vi "plot_normal.vi"(0 "mean":dbl, 1 "standard deviation":dbl, 2 "variance":dbl, 5 "error in (no error)":errorcluster, 6 "xsup":dbl, 8 "xinf":dbl, 10 "N":u16) -> (14 "Normal_xy":cluster{dbl[], dbl[]}, 15 "x":dbl[](array[numeric]), 16 "Normal curve":dbl[](array[numeric]), 19 "error out":errorcluster)   [LabVIEW 2019]
panel:
  in  "Tab Control":enum32{"Page 1", "Page 2"}(tab)
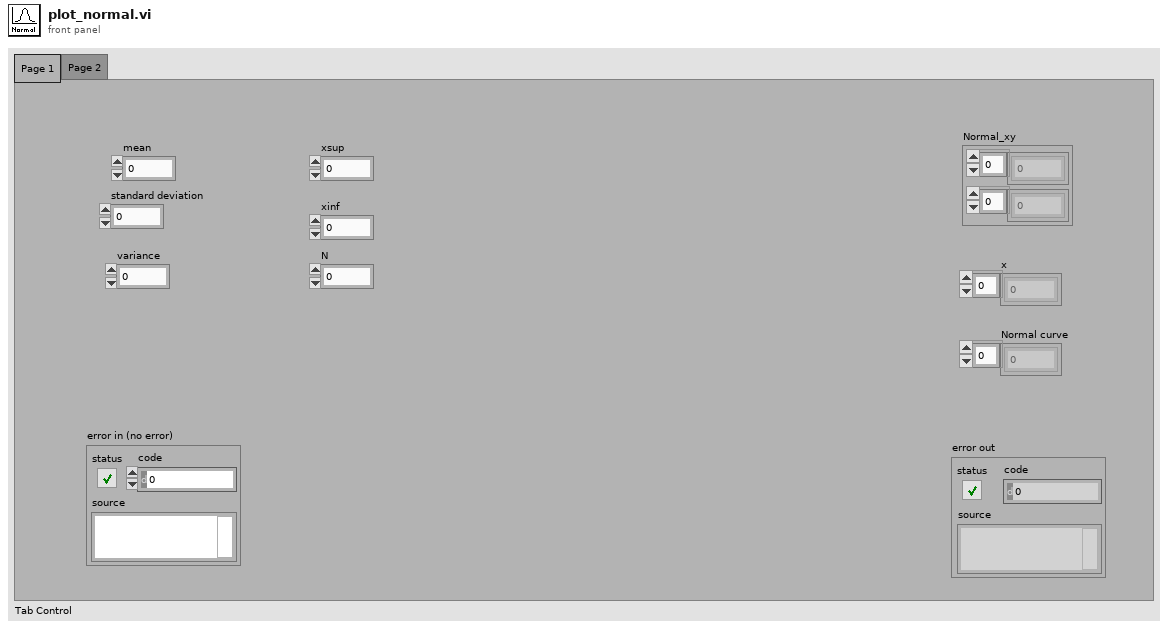
[diagram p1: front panel]
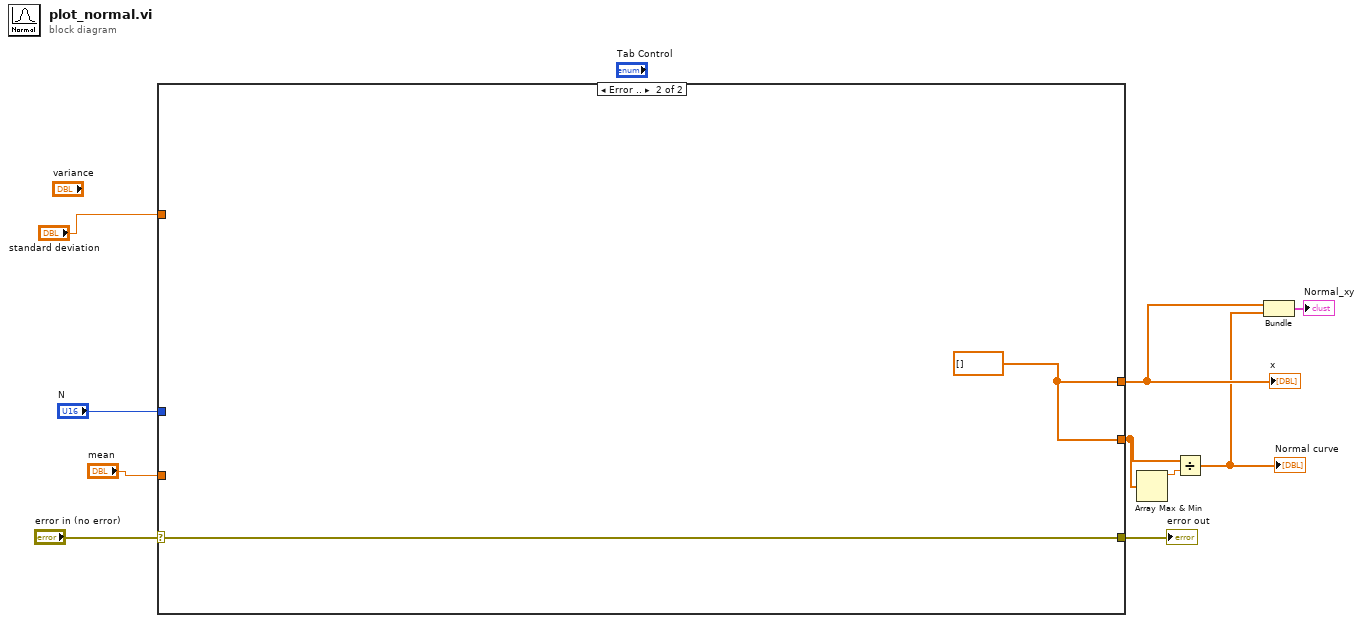
[diagram p0: block diagram]
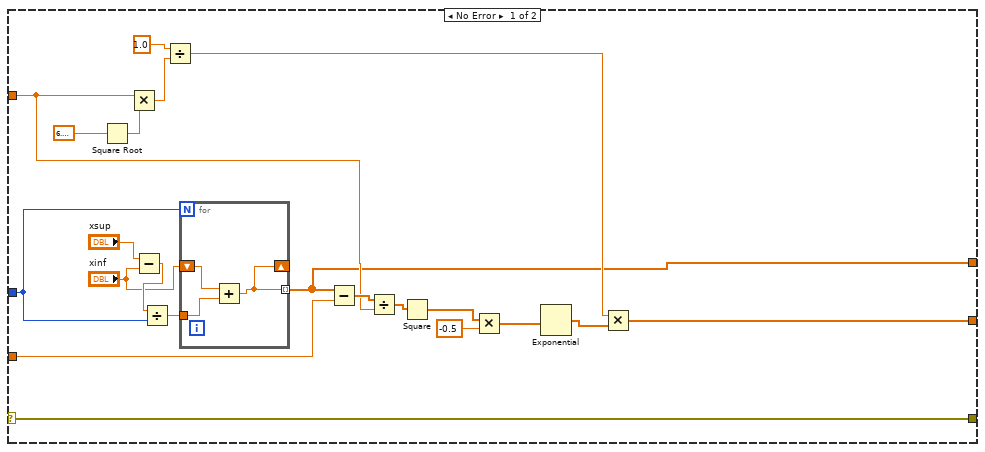
[diagram p2: hidden frame]
diagram:
  n1 = case shown="Error .." "error in (no error)" {
    selector: "error in (no error)" -> [w12 w36]
    tunnel: [w12 w36] -> w10
    tunnel: "N" -> [w31 _]
    tunnel: "standard deviation" -> [w20 _]
    tunnel: "mean" -> [w22 _]
    tunnel: [w13 w35] -> w5
    tunnel: [w11 w35] -> w3
    frame No Error {
      n2 = Square Root(x=6.283185307179586) -> (sqrt(x)=w24:dbl)
      n3 = Multiply(x=w20, y=w24) -> (x*y=w23:dbl)
      n4 = Subtract(x="xsup", y="xinf") -> (x-y=w29:dbl)
      n5 = Divide(x=w29, y=w31) -> (x/y=w28:dbl)
      n6 = Divide(x=1.0, y=w23) -> (x/y=w14:dbl)
      n7 = for {
        N: w31 -> [_]
        tunnel: w28 -> [w34]
        tunnel: [w32] -> w11 mode=indexing
        shift-right: [w32] -> _
        shift-left: "xinf" -> [w33]
        n8 = Add(x=w33, y=w34) -> (x+y=w32:dbl)
      }
      n9 = Subtract(x=w11, y=w22) -> (x-y=w21:dbl[])
      n10 = Divide(x=w21, y=w20) -> (x/y=w18:dbl[])
      n11 = Square(x=w18) -> (x^2=w17:dbl[])
      n12 = Multiply(x=w17, y=-0.5) -> (x*y=w16:dbl[])
      n13 = Exponential(1:w16) -> (0:w15:dbl[])
      n14 = Multiply(x=w14, y=w15) -> (x*y=w13:dbl[])
    }
    frame Error {
      w35 = dbl[] []
    }
  }
  "error out" <- w10
  "x" <- w3
  n15 = Array Max & Min(array=w5) -> (max value=w4:dbl)  [unwired: 3 out]
  n16 = Divide(x=w5, y=w4) -> (x/y=w2:dbl[])
  "Normal curve" <- w2
  n17 = Bundle(w3, w2) -> (→"Normal_xy":cluster{dbl[], dbl[]})  [unwired: 1 in]
